vi "Seven 8-bit Port Digital Input.vi"(2 "Seven 8-bit DI Ports":T1={"8-bit DI Port 0"="Chassis1/Mod4/DI7:0", "8-bit DI Port 1"="Chassis1/Mod4/DI7:0", "8-bit DI Port 2"="Chassis1/Mod4/DI7:0", "8-bit DI Port 3"="Chassis1/Mod4/DI7:0", "8-bit DI Port 4"="Chassis1/Mod4/DI7:0", "8-bit DI Port 5"="Chassis1/Mod4/DI7:0", "8-bit DI Port 6"="Chassis1/Mod4/DI7:0"}) -> (7 "Packet":u64)   [LabVIEW 2009]
uses:
  <vilib>/eio/EIONode/EIONode.xnode
  <vilib>/rvi/eio/nirviEIOImplementation/nirviEIOImplementation.xnode
  <vilib>/rvi/eio/common/nirviEmuTemplateMethod_noerrors.vi
  <vilib>/rvi/eio/common/nirviEmuClasses.ctl
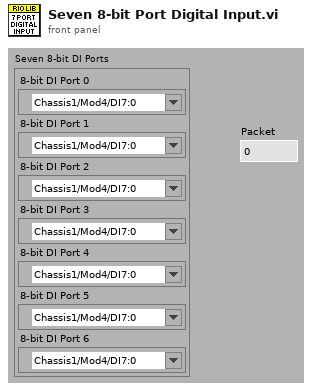
[diagram p1: front panel]
types:
  T1 = cluster{"8-bit DI Port 0":refnum<k21>, "8-bit DI Port 1":refnum<k21>, "8-bit DI Port 2":refnum<k21>, "8-bit DI Port 3":refnum<k21>, "8-bit DI Port 4":refnum<k21>, "8-bit DI Port 5":refnum<k21>, "8-bit DI Port 6":refnum<k21>}
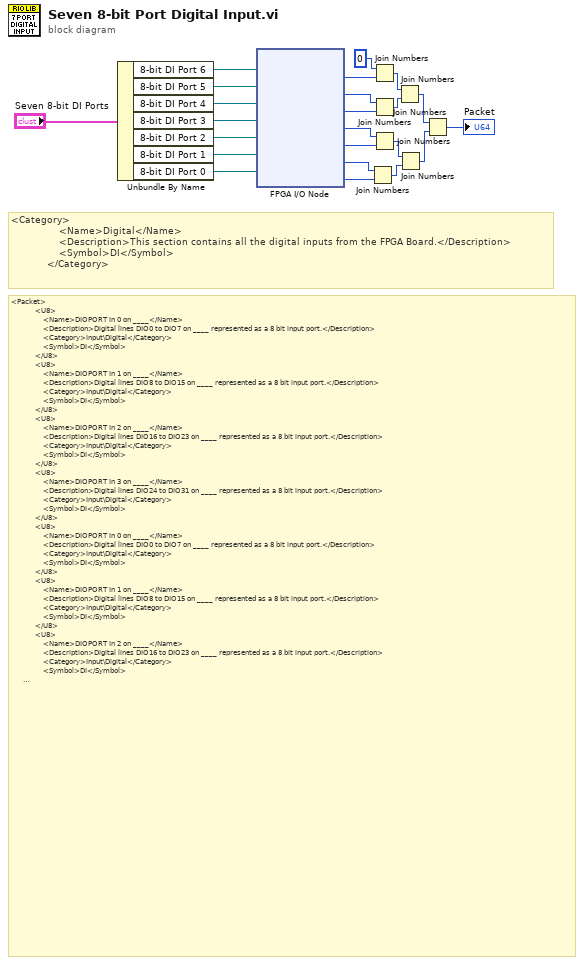
[diagram p0: block diagram]
diagram:
  # "<Packet>\n            <U8>\n                <Name>DIOPORT In 0 on ____</Name>\n                <Description>Digital lines DIO0 to DIO7 on ____ represented as a 8 bit input port.</Description>\n                <Category>Input\\Digital</Category>\n                <Symbol>DI</Symbol>\n            </U8>\n            <U8>\n                <Name>DIOPORT In 1 on ____</Name>\n                <Description>Digital lines DIO8 to DIO15 on ____ represented as a 8 bit input port.</Description>\n                <Category>Input\\Digital</Category>\n                <Symbol>DI</Symbol>\n            </U8>\n            <U8>\n                <Name>DIOPORT In 2 on ____</Name>\n                <Description>Digital lines DIO16 to DIO23 on ____ represented as a 8 bit input port.</Description>\n                <Category>Input\\Digital</Category>\n                <Symbol>DI</Symbol>\n            </U8>\n            <U8>\n                <Name>DIOPORT In 3 on ____</Name>\n                <Description>Digital lines DIO24 to DIO31 on ____ represented as a 8 bit input port.</Description>\n                <Category>Input\\Digital</Category>\n                <Symbol>DI</Symbol>\n            </U8>\n            <U8>\n                <Name>DIOPORT In 0 on ____</Name>\n                <Description>Digital lines DIO0 to DIO7 on ____ represented as a 8 bit input port.</Description>\n                <Category>Input\\Digital</Category>\n                <Symbol>DI</Symbol>\n            </U8>\n            <U8>\n                <Name>DIOPORT In 1 on ____</Name>\n                <Description>Digital lines DIO8 to DIO15 on ____ represented as a 8 bit input port.</Description>\n                <Category>Input\\Digital</Category>\n                <Symbol>DI</Symbol>\n            </U8>\n            <U8>\n                <Name>DIOPORT In 2 on ____</Name>\n                <Description>Digital lines DIO16 to DIO23 on ____ represented as a 8 bit input port.</Description>\n                <Category>Input\\Digital</Category>\n                <Symbol>DI</Symbol>\n            </U8>\n        </Packet>"
  # "<Category>\n                <Name>Digital</Name>\n                <Description>This section contains all the digital inputs from the FPGA Board.</Description>\n                <Symbol>DI</Symbol>\n            </Category>"
  n1 = Unbundle By Name("Seven 8-bit DI Ports") -> ("8-bit DI Port 6"=w5:refnum<k21>, "8-bit DI Port 5"=w7:refnum<k21>, "8-bit DI Port 4"=w10:refnum<k21>, "8-bit DI Port 3"=w12:refnum<k21>, "8-bit DI Port 2"=w16:refnum<k21>, "8-bit DI Port 1"=w18:refnum<k21>, "8-bit DI Port 0"=w19:refnum<k21>)
  n2 = xnode "FPGA I/O Node"("FPGA I/O In"=w5, "FPGA I/O In"=w7, "FPGA I/O In"=w10, "FPGA I/O In"=w12, "FPGA I/O In"=w16, "FPGA I/O In"=w18, "FPGA I/O In"=w19) -> ("I/O Item"=w3:u8, "I/O Item"=w6:u8, "I/O Item"=w8:u8, "I/O Item"=w11:u8, "I/O Item"=w14:u8, "I/O Item"=w17:u8, "I/O Item"=w22:u8)  [unwired: 7 out]
  n3 = Join Numbers(hi=w17, lo=w22) -> ((hi.lo)=w15:u16)
  n4 = Join Numbers(hi=u8 0, lo=w3) -> ((hi.lo)=w1:u16)
  n5 = Join Numbers(hi=w6, lo=w8) -> ((hi.lo)=w4:u16)
  n6 = Join Numbers(hi=w11, lo=w14) -> ((hi.lo)=w13:u16)
  n7 = Join Numbers(hi=w1, lo=w4) -> ((hi.lo)=w9:u32)
  n8 = Join Numbers(hi=w13, lo=w15) -> ((hi.lo)=w23:u32)
  n9 = Join Numbers(hi=w9, lo=w23) -> ((hi.lo)=→"Packet":u64)
